vi "Get Path Loss from s2p File.vi"(8 "error in (no error)":errorcluster, 9 "Frequency (MHz)":dbl=600.0, 10 "Path Name":string, 11 "Calibration Root Directory":path) -> (0 "error out":errorcluster, 2 "Closest Frequency (MHz)":dbl, 3 "Path Loss (dB)":dbl)   [LabVIEW 2025, in "Calibration.lvlib"]
uses:
  Calibration.lvlib
  <vilib>/Utility/error.llb/Error Cluster From Error Code.vi
  <vilib>/Utility/file.llb/Read Delimited Spreadsheet (DBL).vi
  <vilib>/ErrorRing/Error Ring.xnode
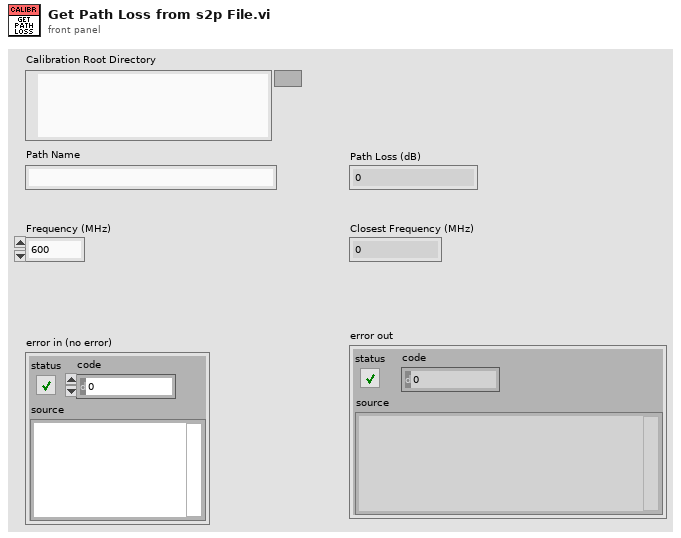
[diagram p1: front panel]
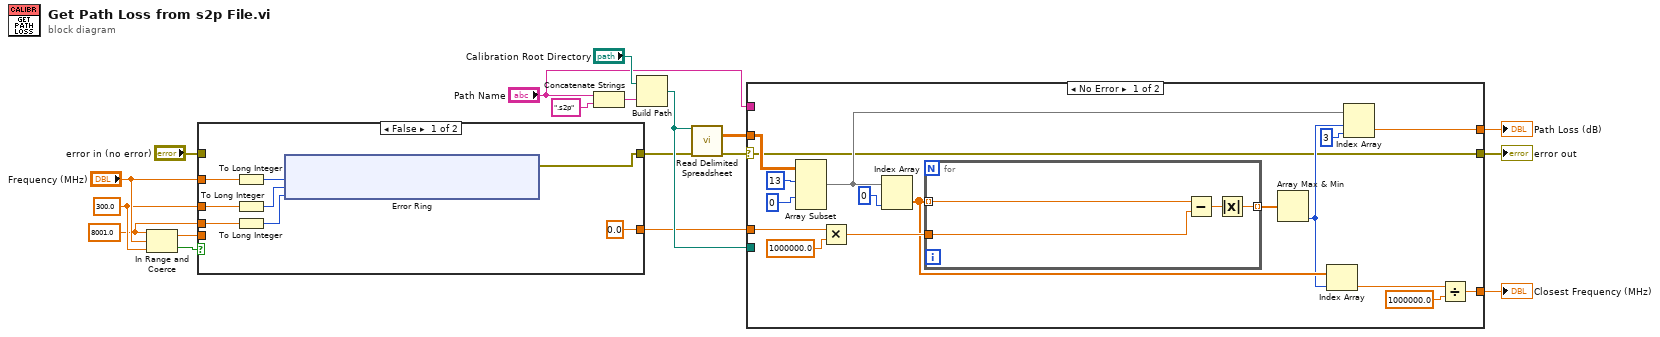
[diagram p0: block diagram]
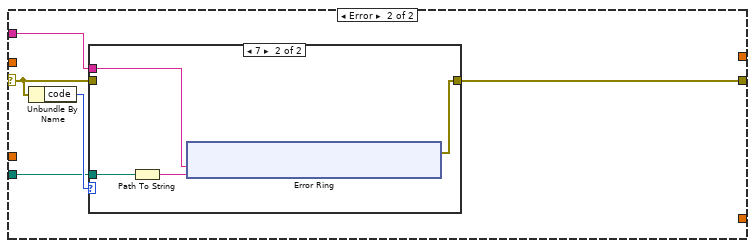
[diagram p3: hidden frame]
diagram:
  w4 = 300.0 ("lower limit")
  w3 = 8001.0 ("upper limit")
  n1 = In Range and Coerce(upper limit=w3, x="Frequency (MHz)", lower limit=w4) -> (coerced(x)=w2:dbl, In Range?=w1:bool)
  n2 = case shown="False" w1 {
    tunnel: [0.0 ("upper limit") w37] -> w7
    tunnel: w2 -> [_ w37]
    tunnel: "error in (no error)" -> [_ w36]
    tunnel: [w25 w36] -> w8
    tunnel: w3 -> [w24 _]
    tunnel: w4 -> [w23 _]
    tunnel: "Frequency (MHz)" -> [w19 _]
    frame False {
      n3 = To Long Integer(number=w19) -> (32bit integer=w20:i32)
      n4 = To Long Integer(number=w23) -> (32bit integer=w21:i32)
      n5 = To Long Integer(number=w24) -> (32bit integer=w22:i32)
      n6 = xnode "Error Ring"("parameter 0"=w20, "parameter 1"=w21, "parameter 2"=w22) -> ("error out"=w25:errorcluster)
    }
    frame True {
    }
  }
  n7 = Concatenate Strings("Path Name", ".s2p") -> (w13:string)
  n8 = Build Path(base path="Calibration Root Directory", name or relative path=w13) -> (appended path=w9:path)
  n9 = call-poly <vilib>:"Read Delimited Spreadsheet.vi"("file path (dialog if empty)"=w9, "error in (no error)"=w8) -> ("all rows"=w18:dbl[][], "error out"=w12:errorcluster)  [unwired: 8 in, 4 out]
  n10 = case shown="No Error" w12 {
    selector: w12 -> [w39 w61]
    tunnel: w18 -> [w54 _]
    tunnel: [w45 _] -> w17
    tunnel: [w40 _] -> w16
    tunnel: [w39 w62] -> w11
    tunnel: "Path Name" -> [_ w60]
    tunnel: w9 -> [_ w59]
    tunnel: w7 -> [w38 _]
    frame No Error {
      n11 = Array Subset(array=w54, index (row)=13 ("index"), index (col)=0 ("index")) -> (w47:dbl[][])  [unwired: 2 in]
      n12 = Multiply(x=w38, y=1000000.0) -> (x*y=w49:dbl)
      n13 = Index Array(array=w47, index (col)=0) -> (element=w44:dbl[])  [unwired: 1 in]
      n14 = for {
        tunnel: w44 -> [w58] mode=indexing
        tunnel: w49 -> [w57]
        tunnel: [w55] -> w48 mode=indexing
        n15 = Subtract(x=w58, y=w57) -> (x-y=w56:dbl)
        n16 = Absolute Value(x=w56) -> (abs(x)=w55:dbl)
      }
      n17 = Array Max & Min(array=w48) -> (min index (indices)=w43:i32)  [unwired: 3 out]
      n18 = Index Array(array=w44, index=w43) -> (element=w42:dbl)
      n19 = Index Array(array=w47, index (row)=w43, index (col)=3) -> (element=w45:dbl)
      n20 = Divide(x=w42, y=1000000.0) -> (x/y=w40:dbl)
    }
    frame Error {
      n21 = Unbundle By Name(w61) -> ("code"=w63:i32)
      n22 = case shown="7" w63 {
        tunnel: [w64 w65] -> w62
        tunnel: w61 -> [w64 _]
        tunnel: w60 -> [_ w68]
        tunnel: w59 -> [_ w67]
        frame 0, Default {
        }
        frame 7 {
          n23 = Path To String(path=w67) -> (string=w66:string)
          n24 = xnode "Error Ring"("parameter 0"=w68, "parameter 1"=w66) -> ("error out"=w65:errorcluster)
        }
      }
    }
  }
  "error out" <- w11
  "Path Loss (dB)" <- w17
  "Closest Frequency (MHz)" <- w16
